vi "SetData.vi"(8 "error in (no error)":errorcluster, 10 "Data":dbl, 11 "ChildSink in":refnum<class "ChildSink.lvclass">) -> (0 "error out":errorcluster, 3 "ChildSink out":refnum<class "ChildSink.lvclass">)   [LabVIEW 2023, in "ChildSink.lvclass"]
uses:
  ChildSink.lvclass
  ChildSink.lvclass/ChildSink.ctl
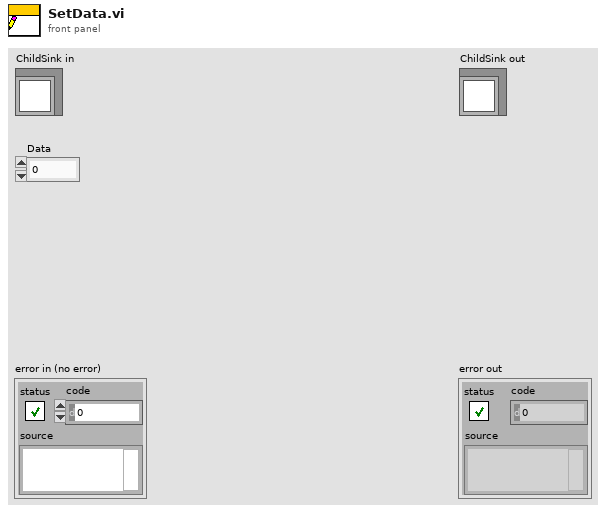
[diagram p1: front panel]
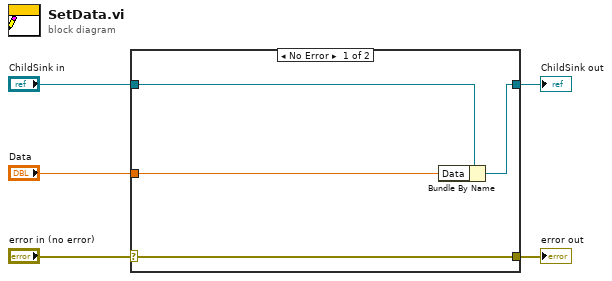
[diagram p0: block diagram]
diagram:
  n1 = case shown="No Error" "error in (no error)" {
    selector: "error in (no error)" -> [w9 w10]
    tunnel: [w9 w10] -> w4
    tunnel: [w7 w11] -> w2
    tunnel: "ChildSink in" -> [w8 w11]
    tunnel: "Data" -> [w6 _]
    frame No Error {
      n2 = Bundle By Name(cluster=w8, "Data"=w6) -> (w7:refnum<class "ChildSink.lvclass">)
    }
    frame Error {
    }
  }
  "error out" <- w4
  "ChildSink out" <- w2
